vi "y16_preview_stop.vi"(5 "COM":bool, 7 "VISA name":refnum<visa-resource-name>, 11 "byPath":u8) -> (3 "return":i32)   [LabVIEW 2016]
panel:
  in  "tVdCmdHeader":T1
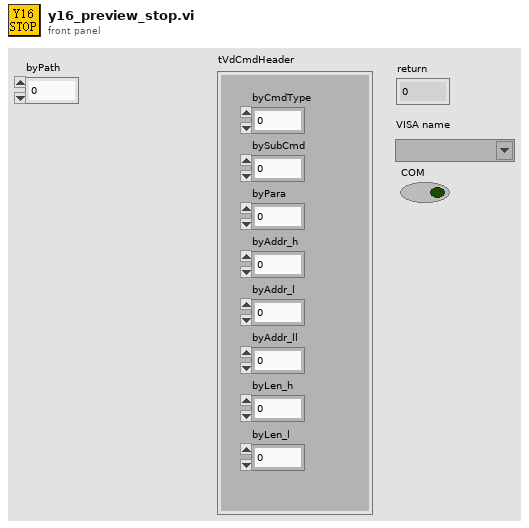
[diagram p1: front panel]
types:
  T1 = cluster{"byCmdType":u8, "bySubCmd":u8, "byPara":u8, "byAddr_h":u8, "byAddr_l":u8, "byAddr_ll":u8, "byLen_h":u8, "byLen_l":u8}
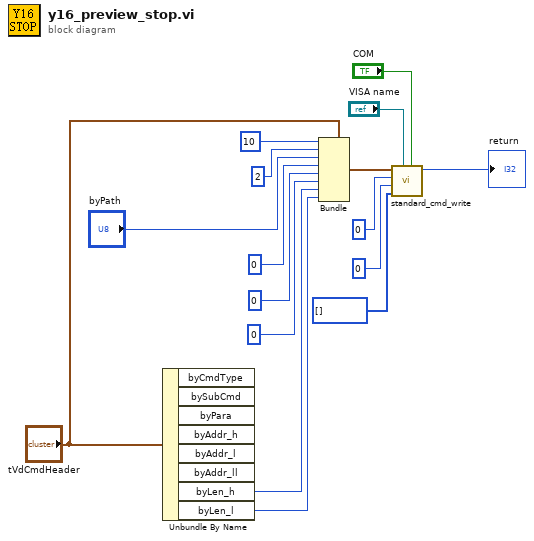
[diagram p0: block diagram]
diagram:
  n1 = Unbundle By Name("tVdCmdHeader") -> ("byLen_h"=w10:u8, "byLen_l"=w9:u8)  [unwired: 6 out]
  n2 = Bundle(cluster="tVdCmdHeader", "byCmdType"=u8 10, "bySubCmd"=u8 2, "byPara"="byPath", "byAddr_h"=u8 0, "byAddr_l"=u8 0, "byAddr_ll"=u8 0, "byLen_h"=w10, "byLen_l"=w9) -> (w8:T1)
  n3 = call "standard_cmd_write.vi"("COM"="COM", "VISA name"="VISA name", "data"=u8[] [], "dwLen"=u32 0, "dwAddr"=u32 0, "cmd_std_header_t"=w8) -> ("return"=→"return":i32)  [unwired: 5 in]
